vi "aimHorizontal.vi"() -> (2 "Done":bool)   [LabVIEW 2012]
panel:
  in  "Speed":dbl=0.2
  in  "deadBand":dbl=1.0
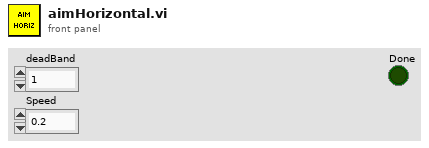
[diagram p1: front panel]
types:
  T1 = typedef "TargetData.ctl" = cluster{"X":dbl, "Y":dbl, "Z":dbl}
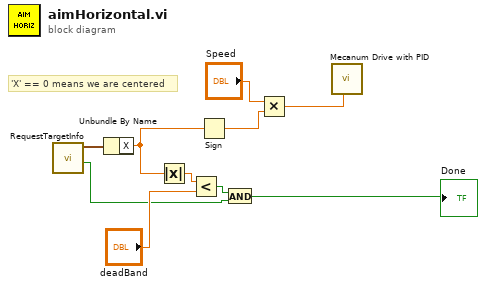
[diagram p0: block diagram]
diagram:
  # "'X' == 0 means we are centered"
  n1 = call "RequestTargetInfo.vi"() -> ("haveInfo"=w6:bool, "Location"=w10:T1)  [unwired: 10 in]
  n2 = Unbundle By Name(w10) -> ("X"=w4:dbl)
  n3 = Absolute Value(x=w4) -> (abs(x)=w9:dbl)
  n4 = Less?(x=w9, y="deadBand") -> (x < y?=w7:bool)
  n5 = Sign(1:w4) -> (0:w3:dbl)
  n6 = And(x=w7, y=w6) -> (x .and. y?=→"Done":bool)
  n7 = Multiply(x="Speed", y=w3) -> (x*y=w1:dbl)
  n8 = call "Mecanum Drive with PID.vi"("Rotation"=w1) -> ()  [unwired: 11 in]
